vi "S3859061_Task2.vi"() -> ()   [LabVIEW 2020]
panel:
  out "count":dbl
  in  "Boolean":bool
  in  "stop":bool
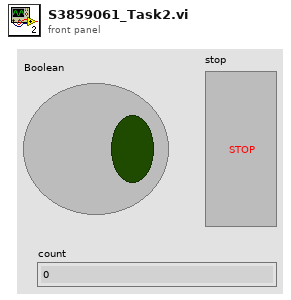
[diagram p1: front panel]
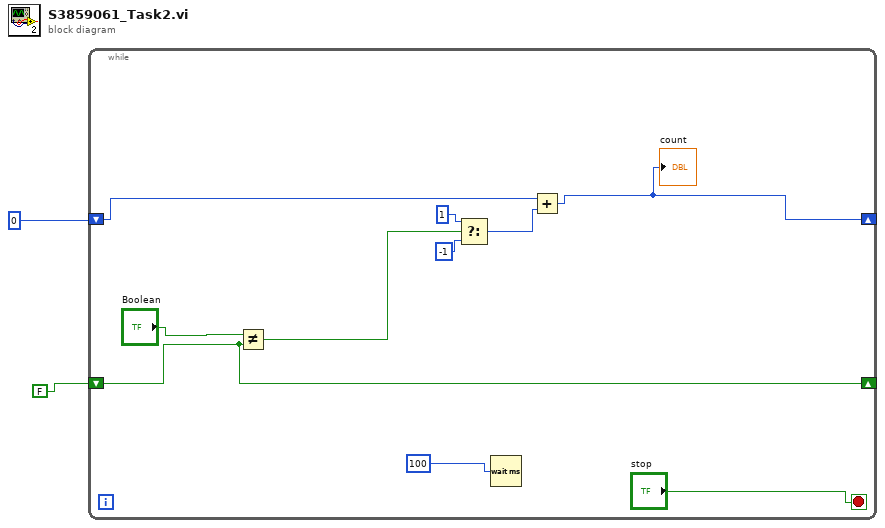
[diagram p0: block diagram]
diagram:
  n1 = while {
    shift-right: [w3] -> _
    shift-left: FALSE -> [w3]
    shift-right: [w5] -> _
    shift-left: 0 -> [w6]
    stop <- "stop" stop-if-true
    n2 = Not Equal?(x="Boolean", y=w3) -> (x != y?=w11:bool)
    n3 = Select(t=1, s=w11, f=-1) -> (s? t:f=w7:i32)
    n4 = Wait (ms)(milliseconds to wait=100) -> ()  [unwired: 1 out]
    n5 = Add(x=w6, y=w7) -> (x+y=w5:i32)
    "count" <- w5
  }
